vi "AIT 1553 - Read incoming message data.vi"(8 "error in (no error)":errorcluster, 10 "Default Msg Data":u16[](array[numeric]), 11 "Driver Data":T1 {"First Word" min=8 max=31; "Num Bits" min=1 max=32; "Start Bit" min=8 max=31}) -> (0 "error out":errorcluster, 3 "Values":dbl[](array[numeric]))   [LabVIEW 2011, in "AIT 1553 Custom Device.lvlib"]
uses:
  AIT 1553 Custom Device.lvlib
  RT Controls/AIT 1553 - Driver Data.ctl
  Controls and Global/Start Bit.ctl
  Controls and Global/Number of Bits.ctl
  System Explorer/Controls/1553 Param.ctl
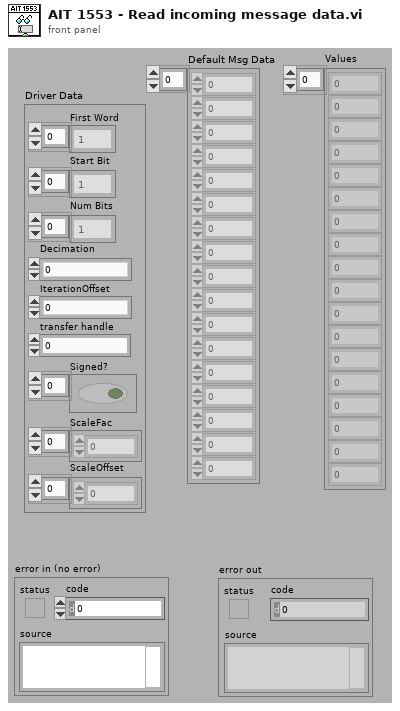
[diagram p1: front panel]
types:
  T1 = typedef "AIT 1553 Custom Device.lvlib/AIT 1553 - Driver Data.ctl" = cluster{"First Word":T2[], "Start Bit":T2[], "Num Bits":T3[], "Decimation":i32, "IterationOffset":i32, "transfer handle":u32, "Signed?":bool[], "ScaleFac":dbl[], "ScaleOffset":dbl[]}
  T2 = typedef "AIT 1553 Custom Device.lvlib/Start Bit.ctl" = i32
  T3 = typedef "AIT 1553 Custom Device.lvlib/Number of Bits.ctl" = i32
  T4 = typedef "AIT 1553 Custom Device.lvlib/1553 Param.ctl" = cluster{"name":string, "firstWord":i32, "startBit":i32, "numberBits":i32, "scaleFactor":dbl, "scaleOffset":dbl, "signed":bool}
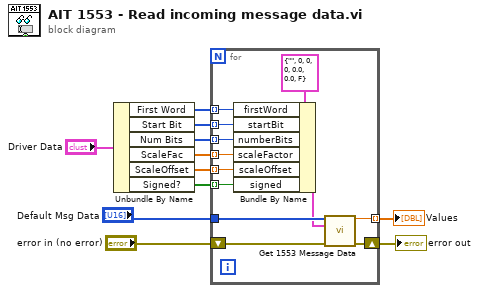
[diagram p0: block diagram]
diagram:
  n1 = Unbundle By Name("Driver Data") -> ("First Word"=w8:T2[], "Start Bit"=w7:T2[], "Num Bits"=w6:T3[], "ScaleFac"=w5:dbl[], "ScaleOffset"=w4:dbl[], "Signed?"=w3:bool[])
  n2 = for {
    tunnel: "Default Msg Data" -> [w23]
    tunnel: w8 -> [w20] mode=indexing
    tunnel: w7 -> [w19] mode=indexing
    tunnel: w6 -> [w18] mode=indexing
    tunnel: w5 -> [w17] mode=indexing
    tunnel: w4 -> [w16] mode=indexing
    tunnel: w3 -> [w15] mode=indexing
    tunnel: [w13] -> w2 mode=indexing
    shift-right: [w12] -> w1
    shift-left: "error in (no error)" -> [w22]
    n3 = Bundle By Name(cluster=T4 {"name"="", "firstWord"=0, "startBit"=0, "numberBits"=0, "scaleFactor"=0.0, "scaleOffset"=0.0, "signed"=FALSE} ("1553 Parameter"), "firstWord"=w20, "startBit"=w19, "numberBits"=w18, "scaleFactor"=w17, "scaleOffset"=w16, "signed"=w15) -> (w14:T4)
    n4 = call "Get 1553 Message Data.vi"("MSG DATA"=w23, "1553 Parameter"=w14, "error in (no error)"=w22) -> ("Value"=w13:dbl, "error out"=w12:errorcluster)  [unwired: 11 in]
  }
  "error out" <- w1
  "Values" <- w2
